vi "ReadInputs.vi"(8 "error in (no error)":errorcluster, 11 "Game in":refnum<class "Game.lvclass">) -> (0 "error out":errorcluster, 3 "Game out":refnum<class "Game.lvclass">)   [LabVIEW 2019, in "RT_Game.lvlib" / "Game.lvclass"]
uses:
  Game.lvclass
  Game.lvclass/Game.ctl
  <vilib>/Utility/error.llb/Error Cluster From Error Code.vi
  <vilib>/rvi/errors/niLvFpgaAdjustHostInterfaceError.vi
  <vilib>/rvi/interface/nirviReadWriteControl/nirviReadWriteControl.xnode
  FPGA_Interface.ctl
  FPGA Bitfiles/myriogameconsole_FPGATarget_Main_ntsPRcBZGxk.lvbitx
  NiFpgaLv.dll
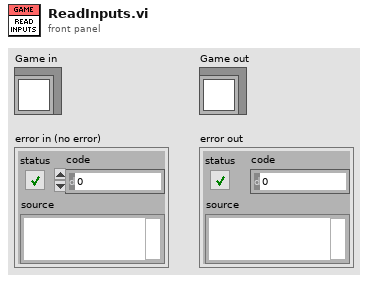
[diagram p1: front panel]
types:
  T1 = typedef "FPGA_Interface.ctl" = refnum<k20>
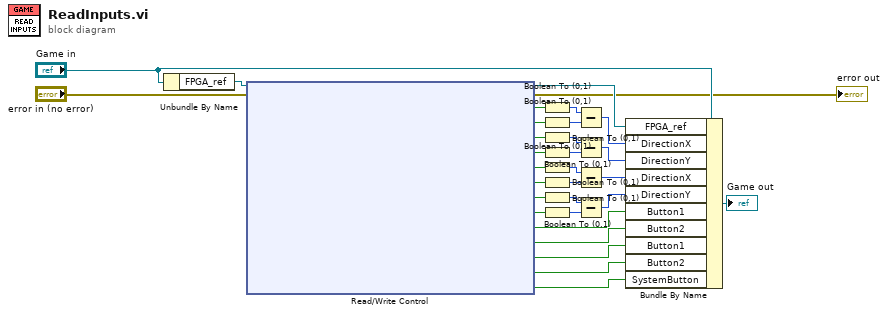
[diagram p0: block diagram]
diagram:
  n1 = Unbundle By Name("Game in") -> ("FPGA_ref"=w28:T1)
  n2 = xnode "Read/Write Control"("FPGA VI Reference In"=w28, "error in"="error in (no error)") -> ("FPGA VI Reference Out"=w10:T1, "error out"=→"error out":errorcluster, "left_right"=w2:bool, "left_left"=w3:bool, "left_down"=w14:bool, "left_up"=w15:bool, "right_right"=w8:bool, "right_left"=w9:bool, "right_down"=w18:bool, "right_up"=w19:bool, "left_1"=w22:bool, "left_2"=w23:bool, "right_1"=w24:bool, "right_2"=w25:bool, "SystemButton"=w27:bool)
  n3 = Boolean To (0,1)(Boolean=w2) -> (0, 1=w4:i16)
  n4 = Boolean To (0,1)(Boolean=w3) -> (0, 1=w5:i16)
  n5 = Boolean To (0,1)(Boolean=w14) -> (0, 1=w13:i16)
  n6 = Boolean To (0,1)(Boolean=w15) -> (0, 1=w12:i16)
  n7 = Boolean To (0,1)(Boolean=w8) -> (0, 1=w7:i16)
  n8 = Boolean To (0,1)(Boolean=w9) -> (0, 1=w6:i16)
  n9 = Boolean To (0,1)(Boolean=w18) -> (0, 1=w26:i16)
  n10 = Boolean To (0,1)(Boolean=w19) -> (0, 1=w17:i16)
  n11 = Subtract(x=w4, y=w5) -> (x-y=w11:i16)
  n12 = Subtract(x=w13, y=w12) -> (x-y=w16:i16)
  n13 = Subtract(x=w7, y=w6) -> (x-y=w20:i16)
  n14 = Subtract(x=w26, y=w17) -> (x-y=w21:i16)
  n15 = Bundle By Name(cluster="Game in", "FPGA_ref"=w10, "DirectionX"=w11, "DirectionY"=w16, "DirectionX"=w20, "DirectionY"=w21, "Button1"=w22, "Button2"=w23, "Button1"=w24, "Button2"=w25, "SystemButton"=w27) -> (→"Game out":refnum<class "Game.lvclass">)
